vi "Test VI Execution Priority.vi"(8 "error in (no error)":errorcluster, 9 "Execution:Priority":T1(ring), 10 "VI Refnum":refnum<vi>, 11 "testStateMachineUtilities in":refnum<class "testStateMachineUtilities.lvclass">) -> (0 "error out":errorcluster, 3 "testStateMachineUtilities out":refnum<class "testStateMachineUtilities.lvclass">)   [LabVIEW 2013]
uses:
  testStateMachineUtilities/testStateMachineUtilities.lvclass
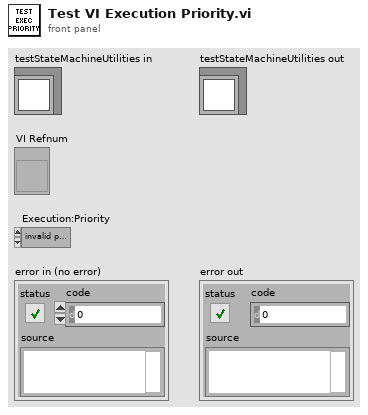
[diagram p1: front panel]
types:
  T1 = enum32{"invalid priority", "background priority", "normal priority", "above normal priority", "high priority", "time critical priority", "subroutine"}
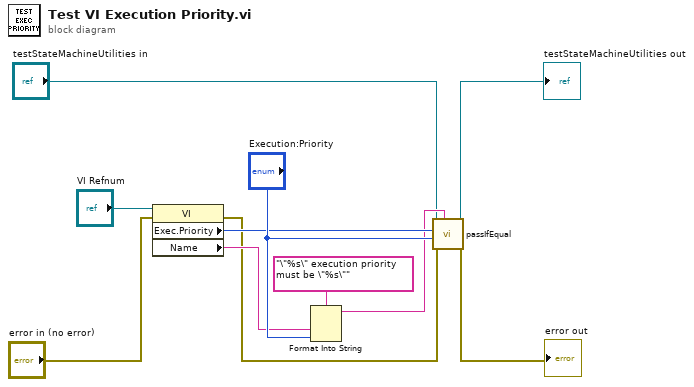
[diagram p0: block diagram]
diagram:
  n1 = property class="VI"(reference="VI Refnum", error in="error in (no error)") -> (error out=w8:errorcluster, "Exec.Priority"=w10:T1, "Name"=w9:string)  [unwired: 1 out]
  n2 = Format Into String(format string="\"%s\" execution priority must be \"%s\"", w9, "Execution:Priority") -> (resulting string=w5:string)  [unwired: 2 in, 1 out]
  n3 = call-dynamic "passIfEqual.vi"("custom report message (\"\")"=w5, "error in (no error)"=w8, "y"="Execution:Priority", "x"=w10, "TestCase in"="testStateMachineUtilities in") -> ("error out"=→"error out":errorcluster, "TestCase out"=→"testStateMachineUtilities out":refnum<class "testStateMachineUtilities.lvclass">)  [unwired: 5 in]
